vi "File System timer.vi"(7 "ctl kind IN 2":T1=enum."set temperature timer", 10 "delta time(sec)":dbl=300.0, 11 "sweep folder path":path) -> (1 "time (min)":dbl)   [LabVIEW 2015]
uses:
  ctl -- name dispatcher -- action.ctl
  next chunk read-write PID -- action.ctl
  file -- 9w path.vi
  array -- find index - real.vi
  array -- interpolate -- i.vi
  ctl -- name dispatcher.vi
  Q -- check range -- i -- real.vi
  Q - not nan -- real.vi
  <vilib>/Utility/libraryn.llb/Check if File or Folder Exists.vi
  file -- read list of lines.vi
  parse -- find first line.vi
  parse -- get list of matches -- numbers.vi
  <vilib>/Utility/file.llb/Write To Spreadsheet File.vi
  <vilib>/Utility/file.llb/Write To Spreadsheet File (string).vi
  <vilib>/gmath/function.llb/Binomial Coefficient.vi
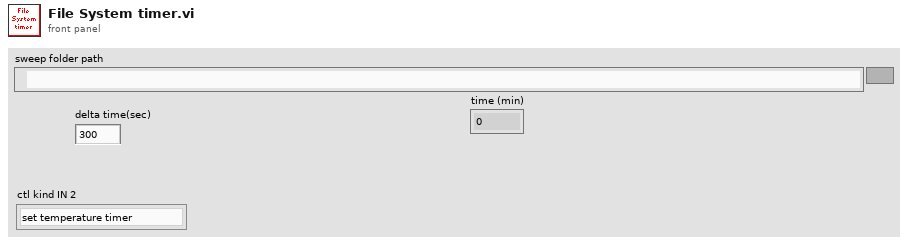
[diagram p1: front panel]
types:
  T1 = typedef "ctl -- name dispatcher -- action.ctl" = enum16{"peak frequency", "peak frequency DUMP", "peak gamma DUMP", "peak gamma", "peak frequency TEST", "peak gamma TEST", "ultrasonic power", "time in gamma", "set temperature ", "set temperature timer", "peak default gamma", "last scan file", "peak freq gamma TEST", "peak NAMES", "errors", "P_I_D", "P", "I", "D", "power vs time", "power vs time TIMER", "void", "power log", "set temperature - SINE", "itc ltc log", "peak - time in gamma"}
  T2 = typedef "next chunk read-write PID -- action.ctl" = enum16{"read", "interpolate", "append col", "write", "write PID col", "append PID col", "interpolate - bezier"}
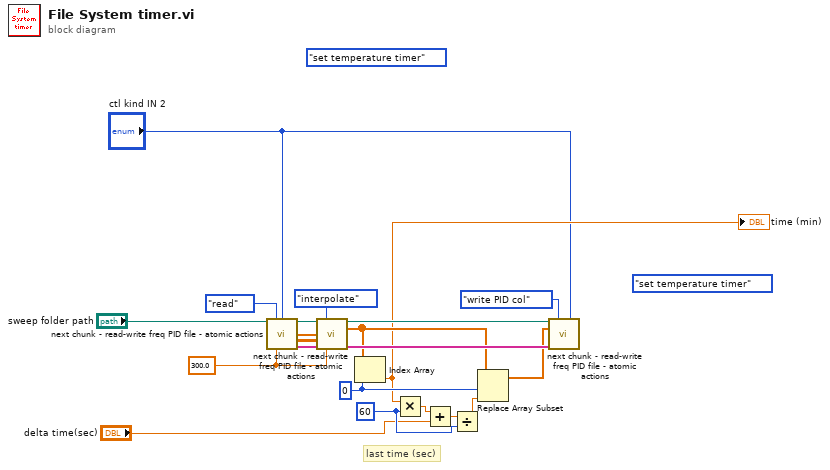
[diagram p0: block diagram]
diagram:
  w4 = 300.0 ("temperature")
  w12 = 0 ("index")
  w7 = 60
  (unwired) ctl_--_name_dispatcher_--_action."set temperature timer" ("ctl kind OUT")
  (unwired) ctl_--_name_dispatcher_--_action."set temperature timer" ("ctl kind IN")
  # "last time (sec)"
  n1 = call "next chunk - read-write freq PID file - atomic actions .vi"("sweep folder path"="sweep folder path", "PID action"=next_chunk_read-write_PID_--_action."read", "ctl kind IN"="ctl kind IN 2", "temperature"=w4) -> ("sweep folder path out"=w18:path, "temperatures"=w16:dbl[], "frequencies"=w15:dbl[][], "header"=w17:string[])  [unwired: 7 in, 1 out]
  n2 = call "next chunk - read-write freq PID file - atomic actions .vi"("PID action"=next_chunk_read-write_PID_--_action."interpolate", "temperatures IN"=w16, "frequencies IN"=w15, "header IN"=w17, "temperature"=w4) -> ("PID freq"=w8:dbl[], "header"=w13:string[])  [unwired: 6 in, 3 out]
  n3 = Index Array(array=w8, index=w12) -> (element=w5:dbl)
  "time (min)" <- w5
  n4 = Multiply(x=w5, y=w7) -> (x*y=w6:dbl)
  n5 = Add(x=w6, y="delta time(sec)") -> (x+y=w10:dbl)
  n6 = Divide(x=w10, y=w7) -> (x/y=w9:dbl)
  n7 = Replace Array Subset(array=w8, new element=w9, index=w12) -> (w11:dbl[])
  n8 = call "next chunk - read-write freq PID file - atomic actions .vi"("sweep folder path"=w18, "PID action"=next_chunk_read-write_PID_--_action."write PID col", "ctl kind OUT"="ctl kind IN 2", "PID freq IN"=w11, "header IN"=w13) -> ()  [unwired: 6 in, 5 out]
